vi "SP Convert Frequency to MHz.vi"(7 "Sweep":T2={"Fstart"=-1.0, "Fstop"=-1.0, "Units"=enum."Hz", "Points"=-1}, 10 "Units":T1=enum."MHz", 11 "Frequency":dbl) -> (3 "Converted Frequency":dbl)   [LabVIEW 2011]
uses:
  TypeDefs/SP Frequency Units.ctl
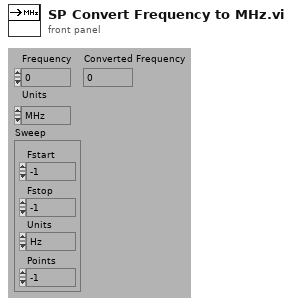
[diagram p1: front panel]
types:
  T1 = typedef "SP Frequency Units.ctl" = enum16{"Hz", "kHz", "MHz", "GHz", "Points"}
  T2 = cluster{"Fstart":dbl, "Fstop":dbl, "Units":T1, "Points":i32}
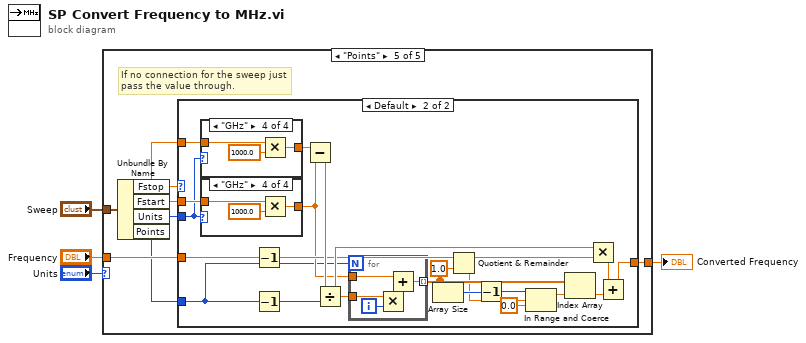
[diagram p0: block diagram]
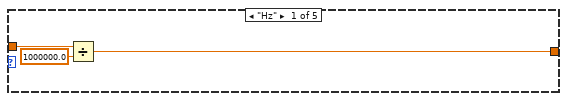
[diagram p2: hidden frame]
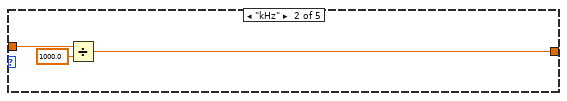
[diagram p3: hidden frame]
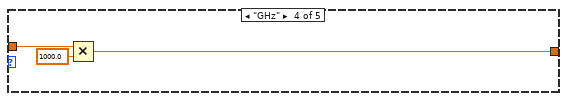
[diagram p5: hidden frame]
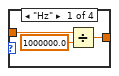
[diagram p7: hidden frame]
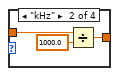
[diagram p8: hidden frame]
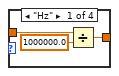
[diagram p10: hidden frame]
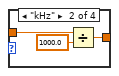
[diagram p11: hidden frame]
diagram:
  n1 = case shown="\"Points\"" "Units" {
    tunnel: "Frequency" -> [w7 w9 w11 w14 w18]
    tunnel: [w6 w8 w11 w13 w16] -> w2
    tunnel: "Sweep" -> [_ _ _ _ w21]
    frame "Hz" {
      n2 = Divide(x=w7, y=1000000.0) -> (x/y=w6:dbl)
    }
    frame "kHz" {
      n3 = Divide(x=w9, y=1000.0) -> (x/y=w8:dbl)
    }
    frame "MHz" {
    }
    frame "GHz" {
      n4 = Multiply(x=w14, y=1000.0) -> (x*y=w13:dbl)
    }
    frame "Points" {
      # "If no connection for the sweep just\npass the value through."
      n5 = Unbundle By Name(w21) -> ("Fstop"=w15:dbl, "Fstart"=w20:dbl, "Units"=w19:T1, "Points"=w17:i32)
      n6 = case shown="Default" w15 {
        tunnel: w15 -> [_ w44]
        tunnel: w20 -> [_ w43]
        tunnel: w19 -> [_ w42]
        tunnel: w18 -> [w22 w40]
        tunnel: w17 -> [_ w29]
        tunnel: [w22 w30] -> w16
        frame -1 {
        }
        frame Default {
          n7 = case shown="\"GHz\"" w42 {
            tunnel: w44 -> [w62 w64 w66 w69]
            tunnel: [w61 w63 w66 w68] -> w41
            frame "Hz" {
              n8 = Divide(x=w62, y=1000000.0) -> (x/y=w61:dbl)
            }
            frame "kHz" {
              n9 = Divide(x=w64, y=1000.0) -> (x/y=w63:dbl)
            }
            frame "MHz", Default {
            }
            frame "GHz" {
              n10 = Multiply(x=w69, y=1000.0) -> (x*y=w68:dbl)
            }
          }
          n11 = case shown="\"GHz\"" w42 {
            tunnel: w43 -> [w52 w54 w56 w59]
            tunnel: [w51 w53 w56 w58] -> w35
            frame "Hz" {
              n12 = Divide(x=w52, y=1000000.0) -> (x/y=w51:dbl)
            }
            frame "kHz" {
              n13 = Divide(x=w54, y=1000.0) -> (x/y=w53:dbl)
            }
            frame "MHz", Default {
            }
            frame "GHz" {
              n14 = Multiply(x=w59, y=1000.0) -> (x*y=w58:dbl)
            }
          }
          n15 = Decrement(x=w40) -> (x-1=w36:dbl)
          n16 = Decrement(x=w29) -> (x-1=w39:i32)
          n17 = Subtract(x=w41, y=w35) -> (x-y=w38:dbl)
          n18 = Divide(x=w38, y=w39) -> (x/y=w37:dbl)
          n19 = for {
            N: w29 -> [_]
            tunnel: w35 -> [w49]
            tunnel: w37 -> [w48]
            tunnel: [w45] -> w28 mode=indexing
            i -> [w47]
            n20 = Multiply(x=w48, y=w47) -> (x*y=w46:dbl)
            n21 = Add(x=w49, y=w46) -> (x+y=w45:dbl)
          }
          n22 = Array Size(array=w28) -> (size(s)=w27:i32)
          n23 = Quotient & Remainder(x=w36, y=1.0) -> (x-y*floor(x/y)=w31:dbl, floor(x/y)=w25:dbl)
          n24 = Decrement(x=w27) -> (x-1=w23:i32)
          n25 = In Range and Coerce(upper limit=w23, x=w25, lower limit=0.0) -> (coerced(x)=w24:dbl)  [unwired: 1 out]
          n26 = Index Array(array=w28, index=w24) -> (element=w33:dbl)
          n27 = Multiply(x=w37, y=w31) -> (x*y=w32:dbl)
          n28 = Add(x=w32, y=w33) -> (x+y=w30:dbl)
        }
      }
    }
  }
  "Converted Frequency" <- w2
